vi "Write.vi"(8 "error in (no error)":errorcluster, 10 "Numeric":dbl, 11 "Numeric Variable in":refnum<class "Double Float.lvclass">) -> (0 "error out":errorcluster, 3 "Numeric Variable out":refnum<class "Double Float.lvclass">)   [LabVIEW 2021, in "Variable.lvlib" / "Double Float.lvclass"]
uses:
  Double Float.lvclass
  Double Float.lvclass/Double Float.ctl
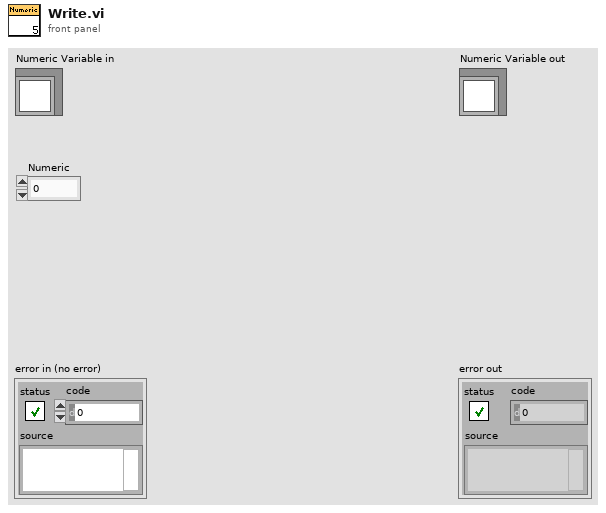
[diagram p1: front panel]
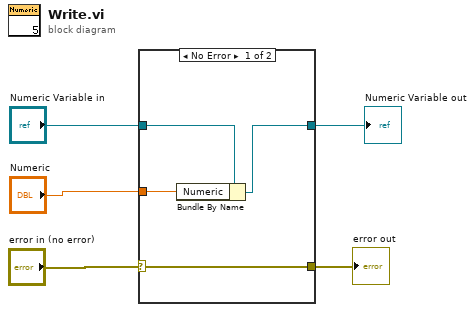
[diagram p0: block diagram]
diagram:
  n1 = case shown="No Error" "error in (no error)" {
    selector: "error in (no error)" -> [w6 w10]
    tunnel: "Numeric Variable in" -> [w9 w11]
    tunnel: "Numeric" -> [w8 _]
    tunnel: [w7 w11] -> w3
    tunnel: [w6 w10] -> w1
    frame No Error {
      n2 = Bundle By Name(cluster=w9, "Numeric"=w8) -> (w7:refnum<class "Double Float.lvclass">)
    }
    frame Error {
    }
  }
  "error out" <- w1
  "Numeric Variable out" <- w3
